vi "GetExperimentCompleted.vi"(11 "Experiment":T1={"File Path"=path "", "Operator"="Operator", "Project"="Project Description", "Target Dose (dpa)"=nan, "Sample"={"Name"="", "Description"="", "Molar Mass (g/mol)"=nan, "Density (g/cm^3)"=nan, "Irradiation Area (cm^2)"=nan, "SRIM Damage Peak (disp * ions/cm)"=nan}, "Beam Line"={"Type"=enum."Ion Beam Analysis", "Ion"=enum."H", "Charge State"=0, "Total Source Ion Energy (kV)"=nan}, "Runs"=[]} {"Beam Line"."Charge State" min=1}) -> (2 "Total Runs":i32, 3 "Experiment Completed (%)":dbl)   [LabVIEW 2012]
uses:
  Experiment.ctl
  Sample.ctl
  BeamLine.ctl
  BeamLineType.ctl
  BeamLineIon.ctl
  ExperimentRun.ctl
  ExperimentRunTiming.ctl
  ExperimentRunDose.ctl
  ExperimentRunFluence.ctl
  ExperimentRunTotalCharge.ctl
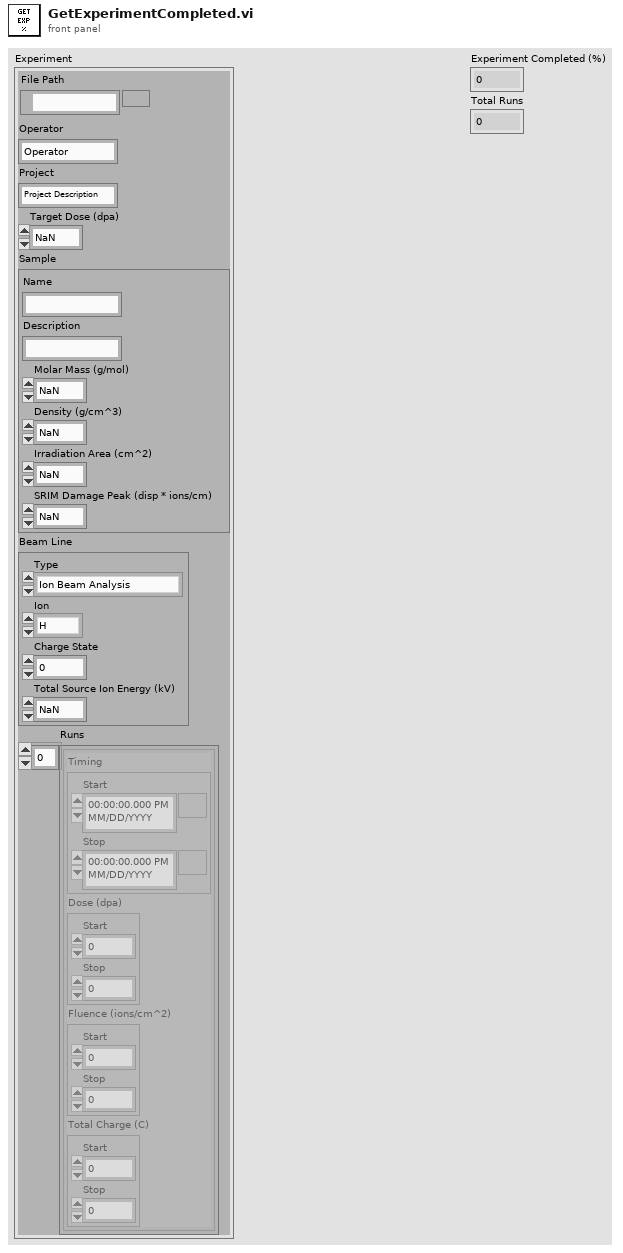
[diagram p1: front panel]
types:
  T1 = typedef "Experiment.ctl" = cluster{"File Path":path, "Operator":string, "Project":string, "Target Dose (dpa)":dbl, "Sample":T2, "Beam Line":T3, "Runs":T6[]}
  T2 = typedef "Sample.ctl" = cluster{"Name":string, "Description":string, "Molar Mass (g/mol)":dbl, "Density (g/cm^3)":dbl, "Irradiation Area (cm^2)":dbl, "SRIM Damage Peak (disp * ions/cm)":dbl}
  T3 = typedef "BeamLine.ctl" = cluster{"Type":T4, "Ion":T5, "Charge State":u8, "Total Source Ion Energy (kV)":dbl}
  T4 = typedef "BeamLineType.ctl" = enum16{"Ion Beam Analysis", "Auxiliary", "Radiation Damage"}
  T5 = typedef "BeamLineIon.ctl" = enum16{"H", "He", "C", "Fe", "Ni", "Pt", "Si", "Ag", "Au"}
  T6 = typedef "ExperimentRun.ctl" = cluster{"Timing":T7, "Dose (dpa)":T8, "Fluence (ions/cm^2)":T9, "Total Charge (C)":T10}
  T7 = typedef "ExperimentRunTiming.ctl" = cluster{"Start":timestamp, "Stop":timestamp}
  T8 = typedef "ExperimentRunDose.ctl" = cluster{"Start":dbl, "Stop":dbl}
  T9 = typedef "ExperimentRunFluence.ctl" = cluster{"Start":dbl, "Stop":dbl}
  T10 = typedef "ExperimentRunTotalCharge.ctl" = cluster{"Start":dbl, "Stop":dbl}
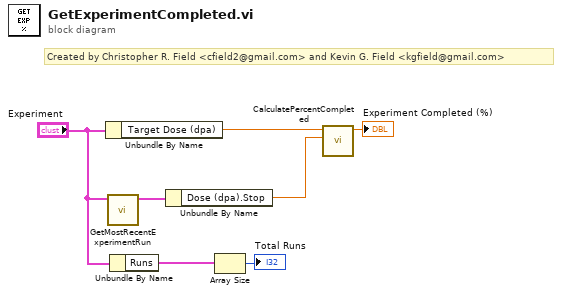
[diagram p0: block diagram]
diagram:
  # "Created by Christopher R. Field <cfield2@gmail.com> and Kevin G. Field <kgfield@gmail.com>"
  n1 = Unbundle By Name("Experiment") -> ("Target Dose (dpa)"=w7:dbl)
  n2 = call "GetMostRecentExperimentRun.vi"("Experiment"="Experiment") -> ("Recent Experiment Run"=w6:T6)  [unwired: 10 in]
  n3 = Unbundle By Name("Experiment") -> ("Runs"=w2:T6[])
  n4 = Unbundle By Name(w6) -> ("Dose (dpa).Stop"=w5:dbl)
  n5 = Array Size(array=w2) -> (size(s)=→"Total Runs":i32)
  n6 = call "CalculatePercentCompleted.vi"("Dose (dpa)"=w5, "Target Dose (dpa)"=w7) -> ("Percent Complete (%)"=→"Experiment Completed (%)":dbl)  [unwired: 8 in, 1 out]
